vi "Get Control Terminal Ref.vi"(0 "Control Reference":refnum<vi>, 1 "error in (no error)":errorcluster) -> (2 "Control Reference Out":refnum<vi>, 3 "Terminal":refnum<vi>, 4 "error out":errorcluster)   [LabVIEW 2018, in "Scripting Tools.lvlib"]
doc: "Get a reference to the terminal corresponding to the control referenced by <B>Control Reference</B>."
uses:
  Scripting Tools.lvlib
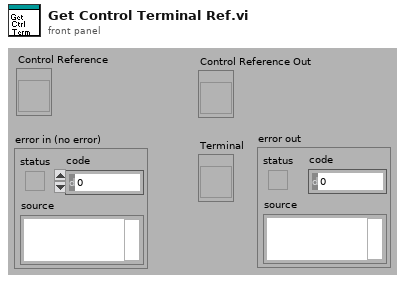
[diagram p1: front panel]
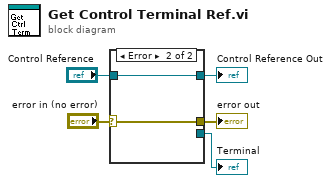
[diagram p0: block diagram]
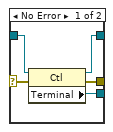
[diagram p2: hidden frame]
diagram:
  n1 = case shown="Error" "error in (no error)" {
    selector: "error in (no error)" -> [w6 w12]
    tunnel: [w10 _] -> w5
    tunnel: [w9 w11] -> w4
    tunnel: "Control Reference" -> [w8 w11]
    tunnel: [w7 w12] -> w2
    frame No Error {
      n2 = property class="Ctl"(reference=w8, error in=w6) -> (reference out=w9:refnum<vi>, error out=w7:errorcluster, "Terminal"=w10:refnum<vi>)
    }
    frame Error {
    }
  }
  "Terminal" <- w5
  "Control Reference Out" <- w4
  "error out" <- w2
